vi "Close.vi"(8 "error in (no error)":errorcluster, 11 "FlexLogger_gRPC in":refnum<class "FlexLogger_gRPC.lvclass">) -> (0 "error out":errorcluster, 3 "FlexLogger_gRPC out":refnum<class "FlexLogger_gRPC.lvclass">)   [LabVIEW 2020, in "FlexLogger_gRPC.lvlib" / "FlexLogger_gRPC.lvclass"]
uses:
  FlexLogger_gRPC.lvclass
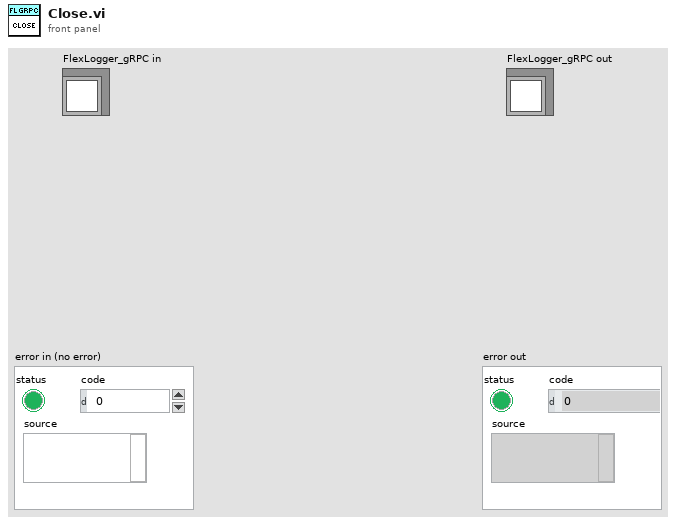
[diagram p1: front panel]
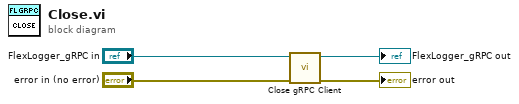
[diagram p0: block diagram]
diagram:
  n1 = call "Close gRPC Client.vi"("error in (no error)"="error in (no error)", "FlexLogger_gRPC in"="FlexLogger_gRPC in") -> ("error out"=→"error out":errorcluster, "FlexLogger_gRPC out"=→"FlexLogger_gRPC out":refnum<class "FlexLogger_gRPC.lvclass">)  [unwired: 8 in]
